vi "Prompt user input.vi"(0 "Enable":bool=TRUE, 1 "String":string, 2 "Parameter Caption":string, 5 "error in (no error)":errorcluster) -> (17 "output":dbl caption="Voltage (V)" format="%#g", 18 "OK":bool, 19 "error out":errorcluster)   [LabVIEW 2020, in "Manual PSU.lvclass"]
doc: "Displays a standard dialog box that prompts users to enter information, such as a user name and password.\n--------------------\n\nThis Express VI is configured as follows:\n\nMessage to Display to the User:Record Voltage Measurement\nThe inputs are: \nNumber: Voltage (V)"
uses:
  Manual PSU.lvclass
panel:
  in  "Voltage (V)":dbl caption="Current (mA)" format="%#g"
  in  "Cancel":bool
  in  "OK2":bool
  in  "OK1":bool
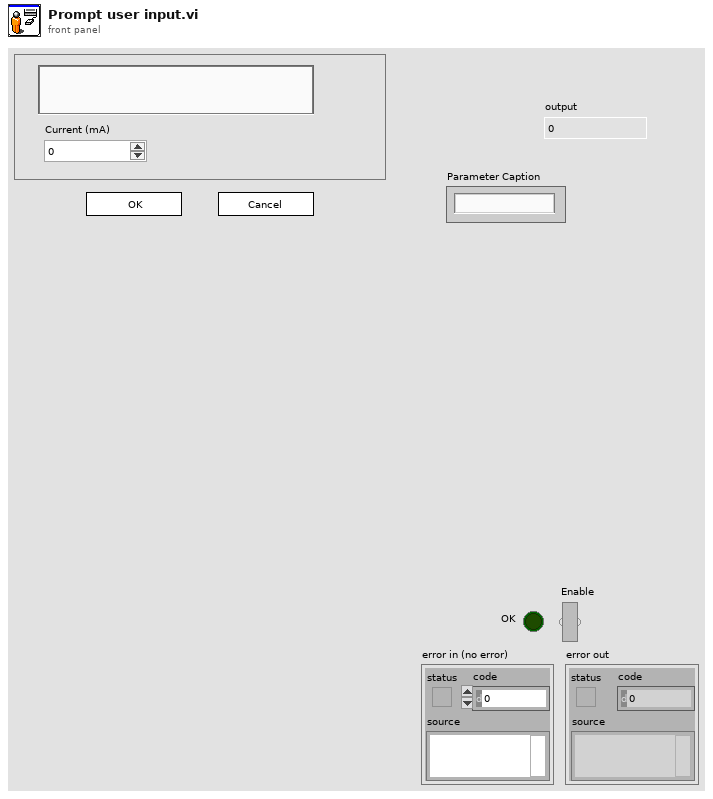
[diagram p1: front panel]
types:
  T1 = cluster{"Input Name":string, "Input Data Type":i32}[]
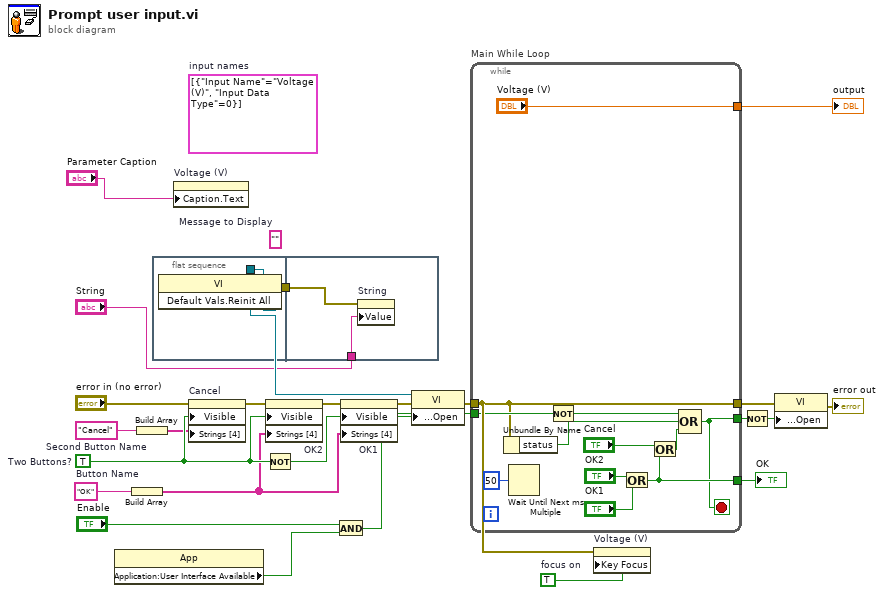
[diagram p0: block diagram]
diagram:
  w5 = TRUE  # focus on
  (unwired) T1 [{"Input Name"="Voltage (V)", "Input Data Type"=0}]  # input names
  w17 = "Cancel"  # Second Button Name
  w15 = "OK"  # Button Name
  (unwired) ""  # Message to Display
  w25 = TRUE  # Two Buttons?
  n1 = property class="App"() -> ("Application:User Interface Available"=w7:bool)  [unwired: 2 in, 2 out]
  n2 = Build Array(w15) -> (w16:string[])
  n3 = Build Array(w17) -> (w18:string[])
  n4 = flat-sequence {
    tunnel: [w27] -> w4
    tunnel: [w26] -> w2
    tunnel: "String" -> [w29]
    tunnel: w2 -> [w28]
    frame #0 {
      n5 = invoke class="VI" method="Default Vals.Reinit All"() -> (reference out=w27:refnum<vi>, error out=w26:errorcluster)  [unwired: 3 in, 1 out]
    }
    frame #1 {
      n6 = property on="String" class="Str"(error in=w28, "Value"=w29) -> ()  [unwired: 1 in, 2 out]
    }
  }
  n7 = property on="Voltage (V)" class="DigNum (strict)"("Caption.Text"="Parameter Caption") -> ()  [unwired: 2 in, 2 out]
  n8 = property on="Cancel" class="Bool"(error in="error in (no error)", "Visible"=w25, "Strings [4]"=w18) -> (error out=w22:errorcluster)  [unwired: 1 in, 1 out]
  n9 = Not(x=w25) -> (.not. x?=w23:bool)
  n10 = property on="OK2" class="Bool"(error in=w22, "Visible"=w25, "Strings [4]"=w16) -> (error out=w21:errorcluster)  [unwired: 1 in, 1 out]
  n11 = And(x="Enable", y=w7) -> (x .and. y?=w8:bool)
  n12 = property on="OK1" class="Bool"(error in=w21, "Visible"=w23, "Strings [4]"=w16) -> (error out=w14:errorcluster)  [unwired: 1 in, 1 out]
  n13 = property class="VI"(reference=w4, error in=w14, "Front Panel Window:Open"=w8) -> (error out=w13:errorcluster)  [unwired: 1 out]
  n14 = while "Main While Loop" {
    tunnel: [w38] -> w24
    tunnel: w8 -> [w36]
    tunnel: [w34] -> w19
    tunnel: w13 -> [w33]
    tunnel: [w33] -> w11
    tunnel: ["Voltage (V)"] -> w6
    stop <- w34 stop-if-true
    n15 = Unbundle By Name(w33) -> ("status"=w31:bool)
    n16 = Wait Until Next ms Multiple(millisecond multiple=u32 50) -> ()  [unwired: 1 out]
    n17 = Not(x=w36) -> (.not. x?=w35:bool)
    n18 = Or(x="OK2", y="OK1") -> (x .or. y?=w38:bool)
    n19 = Or(x="Cancel", y=w38) -> (x .or. y?=w32:bool)
    n20 = Compound Arithmetic op=OR(w35, w31, w32) -> (w34:bool)
  }
  "OK" <- w24
  "output" <- w6
  n21 = property on="Voltage (V)" class="DigNum (strict)"(error in=w13, "Key Focus"=w5) -> ()  [unwired: 1 in, 2 out]
  n22 = Not(x=w19) -> (.not. x?=w20:bool)
  n23 = property class="VI"(error in=w11, "Front Panel Window:Open"=w20) -> (error out=→"error out":errorcluster)  [unwired: 1 in, 1 out]
